vi "_datatypeChecker.vi"(9 "Type":T1, 10 "key":string, 11 "cacher (in)":variant) -> (0 "error out":errorcluster, 1 "stored type":T1, 2 "match?":bool, 3 "cacher":variant)   [LabVIEW 2017, in "TagDB.lvlib"]
uses:
  TagDB.lvlib
  <vilib>/Utility/Data Type/Type Definitions/Data Type.ctl
  <vilib>/Utility/Data Type/NI_Data Type.lvlib
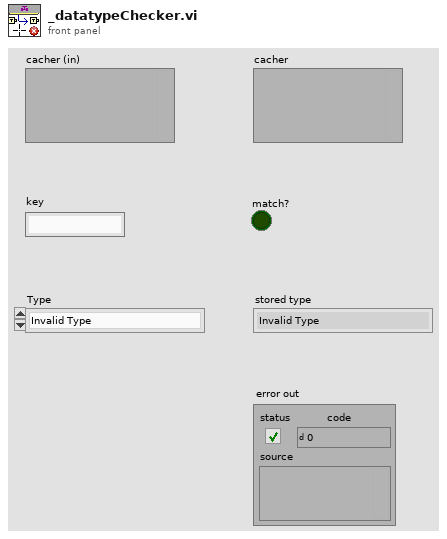
[diagram p1: front panel]
types:
  T1 = typedef "NI_Data Type.lvlib/Data Type.ctl" = enum8{"Invalid Type", "Void", "I8", "I16", "I32", "I64", "U8", "U16", "U32", "U64", "Single Float", "Double Float", "Extended Float", "Single Complex", "Double Complex", "Extended Complex", "Enum U8", "Enum U16", "Enum U32", "Enum U64", "Single Float With Unit", "Double Float With Unit", "Extended Float With Unit", "Single Complex with Unit", "Double Complex with Unit", "Extended Complex with Unit", "Boolean", "String", "Path", "Picture", "Tag", "Array", "Cluster", "Variant", "LV Variant", "Waveform", "Timestamp", "Digital Waveform", "Digital Data", "ExpressData", "Refnum", "External Data", "VI", "Poly VI", "LabVIEW Class Instance", "Fixed Point"}
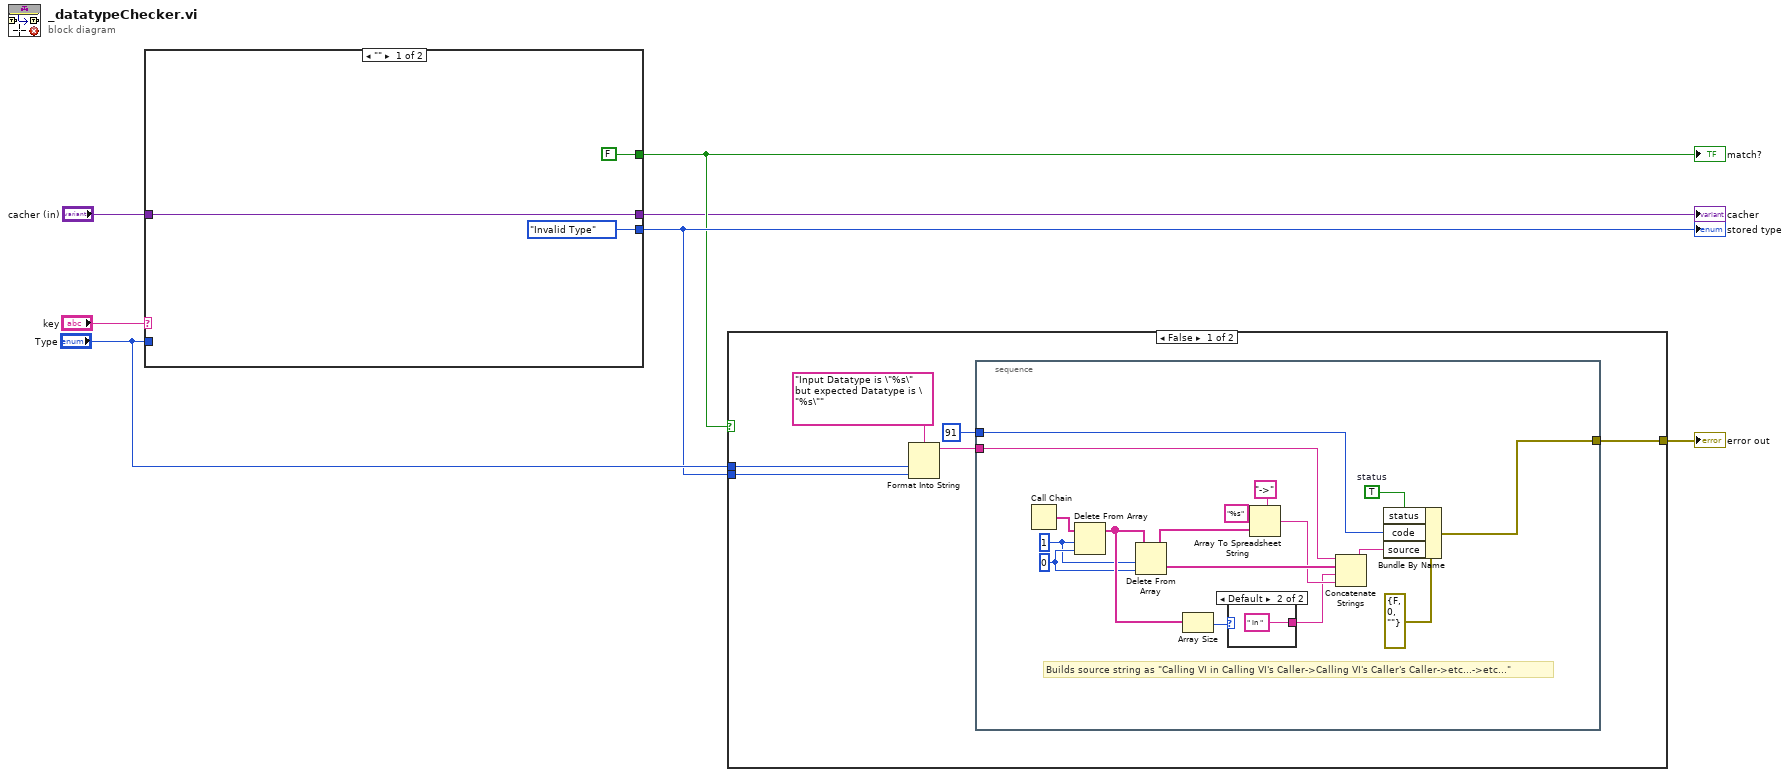
[diagram p0: block diagram]
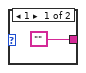
[diagram p2: hidden frame]
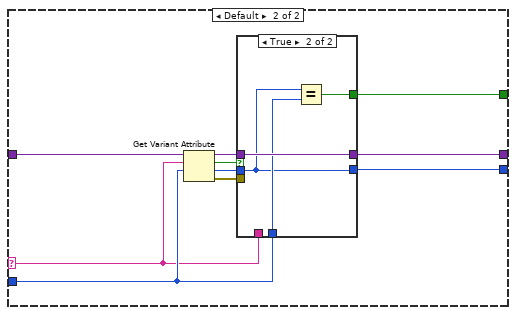
[diagram p4: hidden frame]
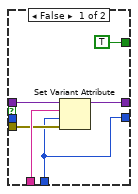
[diagram p5: hidden frame]
diagram:
  n1 = case shown="\"\"" "key" {
    selector: "key" -> [_ w15]
    tunnel: "cacher (in)" -> [w10 w12]
    tunnel: [w10 w11] -> w2
    tunnel: "Type" -> [_ w16]
    tunnel: [FALSE w14] -> w3
    tunnel: [Data_Type."Invalid Type" ("Type") w13] -> w4
    frame "" {
    }
    frame Default {
      n2 = Get Variant Attribute(Variant=w12, name=w15, default value (empty Variant)=w16) -> (duplicate Variant=w20:variant, found=w19:bool, value=w18:T1, error out=w17:errorcluster)  [unwired: 1 in]
      n3 = case shown="True" w19 {
        tunnel: w20 -> [w26 w30]
        tunnel: w15 -> [w25 _]
        tunnel: w18 -> [_ w27]
        tunnel: w17 -> [w24 _]
        tunnel: [w23 w30] -> w11
        tunnel: w16 -> [w21 w29]
        tunnel: [TRUE w28] -> w14
        tunnel: [w21 w27] -> w13
        frame False {
          n4 = Set Variant Attribute(Variant=w26, name=w25, value=w21, error in=w24) -> (Variant out=w23:variant)  [unwired: 2 out]
        }
        frame True {
          n5 = Equal?(x=w27, y=w29) -> (x = y?=w28:bool)
        }
      }
    }
  }
  "cacher" <- w2
  "match?" <- w3
  "stored type" <- w4
  n6 = case shown="False" w3 {
    tunnel: [w36 _] -> w6
    tunnel: "Type" -> [w32 _]
    tunnel: w4 -> [w31 _]
    frame False {
      n7 = Format Into String(format string="Input Datatype is \"%s\" but expected Datatype is \"%s\"", w32, w31) -> (resulting string=w33:string)  [unwired: 2 in, 1 out]
      n8 = stacked-sequence {
        tunnel: [w49] -> w36
        tunnel: w33 -> [w50]
        tunnel: 91 ("code") -> [w46]
        frame #0 {
          w43 = 0 ("Index")
          w42 = 1 ("Length")
          w47 = TRUE  # status
          # "Builds source string as \"Calling VI in Calling VI's Caller->Calling VI's Caller's Caller->etc...->etc...\""
          n9 = Call Chain() -> (call chain=w37:string[])
          n10 = Delete From Array(array=w37, length=w42, index=w43) -> (array with subset deleted=w53:string[])  [unwired: 1 out]
          n11 = Delete From Array(array=w53, length=w42, index=w43) -> (deleted portion=w52:string[], array with subset deleted=w44:string[])
          n12 = Array Size(array=w53) -> (size(s)=w51:i32)
          n13 = case shown="Default" w51 {
            tunnel: ["" " in " ("Format String")] -> w39
            frame 1 {
            }
            frame Default {
            }
          }
          n14 = Array To Spreadsheet String(delimiter (Tab)="->", array=w44, 3:"%s" ("format string")) -> (spreadsheet string=w40:string)
          n15 = Concatenate Strings(w50, w52, w39, w40) -> (w48:string)
          n16 = Bundle By Name(cluster=errorcluster {"status"=FALSE, "code"=0, "source"=""} ("error out"), "status"=w47, "code"=w46, "source"=w48) -> (w49:errorcluster)
        }
      }
    }
    frame True {
    }
  }
  "error out" <- w6
